vi "monitor INTAKE power curve.vi"() -> ()   [LabVIEW 2023]
uses:
  <vilib>/Rock Robotics/WPI/ThirdParty/REV Robotics/REVLib/Typedef/Spark MAX Parameter ID.ctl
  <vilib>/Rock Robotics/WPI/ThirdParty/REV Robotics/REVLib/Typedef/Spark MAX Parameter Type.ctl
  Global INIT.vi
  Global stack names.vi
panel:
  out "motor rpm":dbl
  out "kVelocity\nConversion":dbl
  out "kPosition\nConversion":dbl
  in  "reset maxes":bool
  out "Power (W)\nMAX":dbl format="%#_13g"
  out "current (A)\nMAX":dbl format="%#_13g"
  out "Temp (F)\nMAX":i8
  out "Monitoring INTAKE motor":T1(graph)
  in  "error in (no error)":errorcluster
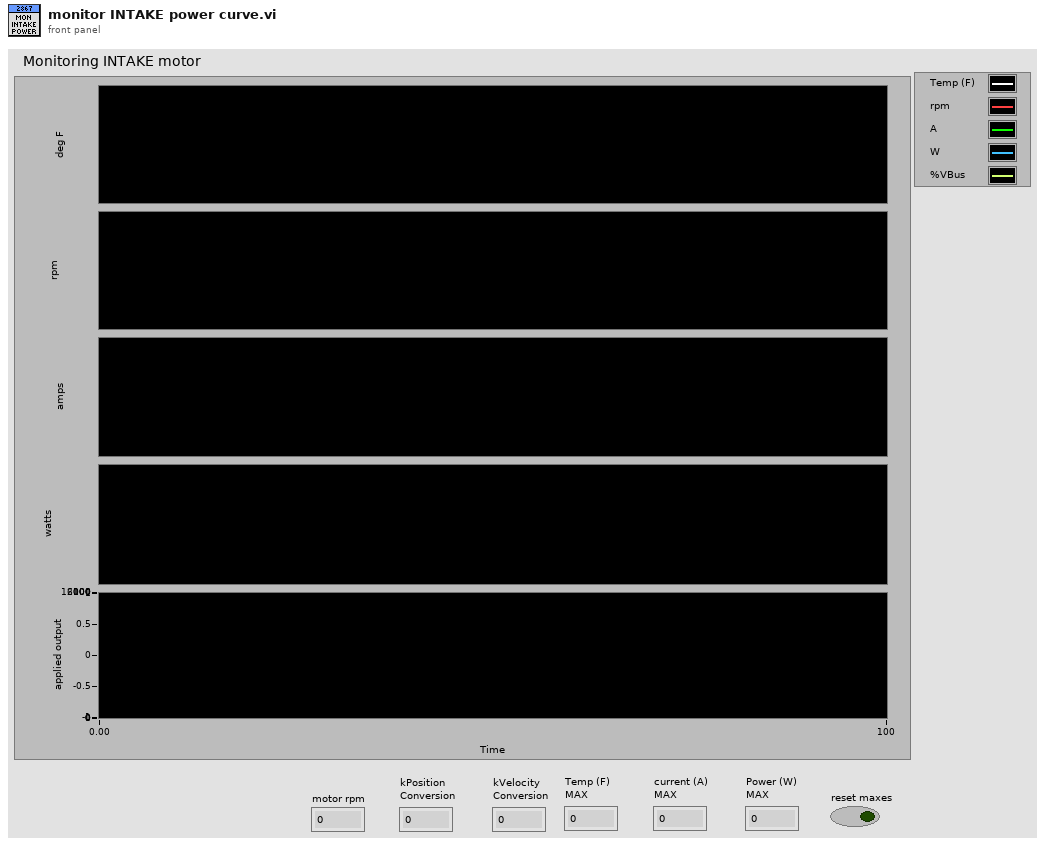
[diagram p1: front panel]
types:
  T1 = cluster{"Motor Temperature":u8, "Sensor Velocity":dbl, "Motor Current":dbl, dbl, "Applied Output":dbl}
  T2 = typedef "Spark MAX Parameter Type.ctl" = enum16{"Signed Int", "Unsigned Int", "Float", "Bool"}
  T3 = typedef "Spark MAX Parameter ID.ctl" = enum16{"kCanID", "kInputMode", "kMotorType", "kCommAdvance", "kSensorType", "kCtrlType", "kIdleMode", "kInputDeadband", "kFeedbackSensorPID0", "kFeedbackSensorPID1", "kPolePairs", "kCurrentChop", "kCurrentChopCycles", "kP_0", "kI_0", "kD_0", "kF_0", "kIZone_0", "kDFilter_0", "kOutputMin_0", "kOutputMax_0", "kP_1", "kI_1", "kD_1", "kF_1", "kIZone_1", "kDFilter_1", "kOutputMin_1", "kOutputMax_1", "kP_2", "kI_2", "kD_2", "kF_2", "kIZone_2", "kDFilter_2", "kOutputMin_2", "kOutputMax_2", "kP_3", "kI_3", "kD_3", "kF_3", "kIZone_3", "kDFilter_3", "kOutputMin_3", "kOutputMax_3", "kInverted", "kOutputRatio", "kSerialNumberLow", "kSerialNumberMid", "kSerialNumberHigh", "kLimitSwitchFwdPolarity", "kLimitSwitchRevPolarity", "kHardLimitFwdEn", "kHardLimitRevEn", "kSoftLimitFwdEn", "kSoftLimitRevEn", "kRampRate", "kFollowerID", "kFollowerConfig", "kSmartCurrentStallLimit", "kSmartCurrentFreeLimit", "kSmartCurrentConfig", "kSmartCurrentReserved", "kMotorKv", "kMotorR", "kMotorL", "kMotorRsvd1", "kMotorRsvd2", "kMotorRsvd3", "kEncoderCountsPerRev", "kEncoderAverageDepth", "kEncoderSampleDelta", "kEncoderInverted", "kEncoderRsvd1", "kClosedLoopVoltageMode", "kCompensatedNominalVoltage", "kSmartMotionMaxVelocity_0", "kSmartMotionMaxAccel_0", "kSmartMotionMinVelOutput_0", "kSmartMotionAllowedClosedLoopError_0", "kSmartMotionAccelStrategy_0", "kSmartMotionMaxVelocity_1", "kSmartMotionMaxAccel_1", "kSmartMotionMinVelOutput_1", "kSmartMotionAllowedClosedLoopError_1", "kSmartMotionAccelStrategy_1", "kSmartMotionMaxVelocity_2", "kSmartMotionMaxAccel_2", "kSmartMotionMinVelOutput_2", "kSmartMotionAllowedClosedLoopError_2", "kSmartMotionAccelStrategy_2", "kSmartMotionMaxVelocity_3", "kSmartMotionMaxAccel_3", "kSmartMotionMinVelOutput_3", "kSmartMotionAllowedClosedLoopError_3", "kSmartMotionAccelStrategy_3", "kIMaxAccum_0", "kSlot3Placeholder1_0", "kSlot3Placeholder2_0", "kSlot3Placeholder3_0", "kIMaxAccum_1", "kSlot3Placeholder1_1", "kSlot3Placeholder2_1", "kSlot3Placeholder3_1", "kIMaxAccum_2", "kSlot3Placeholder1_2", "kSlot3Placeholder2_2", "kSlot3Placeholder3_2", "kIMaxAccum_3", "kSlot3Placeholder1_3", "kSlot3Placeholder2_3", "kSlot3Placeholder3_3", "kPositionConversionFactor", "kVelocityConversionFactor", "kClosedLoopRampRate", "kSoftLimitFwd", "kSoftLimitRev", "kSoftLimitRsvd0", "kSoftLimitRsvd1", "kAnalogPositionConversion", "kAnalogVelocityConversion", "kAnalogAverageDepth", "kAnalogSensorMode", "kAnalogInverted", "kAnalogSampleDelta", "kAnalogRsvd0", "kAnalogRsvd1", "kDataPortConfig", "kAltEncoderCountsPerRev", "kAltEncoderAverageDepth", "kAltEncoderSampleDelta", "kAltEncoderInverted", "kAltEncoderPositionConversion", "kAltEncoderVelocityConversion", "kAltEncoderRsvd0", "kAltEncoderRsvd1", "kHallSensorSampleRate", "kHallSensorAverageDepth", "kNumParameters", "kDutyCyclePositionFactor", "kDutyCycleVelocityFactor", "kDutyCycleInverted", "kDutyCycleSensorMode", "kDutyCycleAverageDepth", "kDutyCycleSampleDelta", "kDutyCycleOffsetv1p6p2", "kDutyCycleRsvd0", "kDutyCycleRsvd1", "kDutyCycleRsvd2", "kPositionPIDWrapEnable", "kPositionPIDMinInput", "kPositionPIDMaxInput", "kDutyCycleZeroCentered", "kDutyCyclePrescalar", "kDutyCycleOffset", "kProductId", "kDeviceMajorVersion", "kDeviceMinorVersion"}
  T4 = typedef "ctrl swerve motor.ctl" = cluster{"description":string, "MOTOR SELECT":T5, "Installed?":bool, "CAN ID":u8, "refnum name":string, "Invert":bool, "Idle Mode":T6, "Current limiting":T7, "MOTOR PIDF coefficients":T8, "gear ratio":dbl}
  T5 = typedef "ctrl MOTOR SELECT.ctl" = i16
  T6 = typedef "Spark MAX Idle Mode.ctl" = enum16{"Coast", "Brake"}
  T7 = typedef "ctrl Spark MAX current limiting.ctl" = cluster{"Linearized":bool, "Free Speed (A)":dbl, "Primay (A)":dbl, "Limit RPM (0)":u32}
  T8 = typedef "ctrl motor PIDF coefficients.ctl" = cluster{"PIDF":cluster{"P Gain":dbl, "I Gain":dbl, "D Gain":dbl, "F Gain":dbl, "I Zone":dbl, "Min Output":dbl, "Max Output":dbl}, "Smart Motion":T9}
  T9 = typedef "Spark MAX Smart Motion Parameters.ctl" = cluster{"Max Velocity":dbl, "Max Acceleration":dbl, "Minimum Velocity Output":dbl, "Allowed Closed Loop Error":dbl}
  T10 = typedef "WPI_MotorControlDeviceRef.ctl" = cluster{"DeviceStatus":errorcluster, "Type":T11, "PWM":cluster{"PWM Channel":T12, "DeadBand":T13}, "CAN":cluster{"Device Number":u8, "SetOutput VI Ref":variant, "GetOutput VI Ref":variant, "Enable VI Ref":variant, "Disable VI Ref":variant, "Data":variant}, "Invert":bool, "DIO PWM":cluster{"PWM \"Enable\" Channel":T12, "DIOChannel":T14, "PWM Rate":dbl}}
  T11 = typedef "WPI_MotorControlType.ctl" = enum16{"PWM", "CAN", "DIO PWM"}
  T12 = typedef "FPGA_DIOPWMChannel.ctl" = enum8{"PWM 0", "PWM 1", "PWM 2", "PWM 3", "PWM 4", "PWM 5", "PWM 6", "PWM 7", "PWM 8", "PWM 9", "PWM MXP 0", "PWM MXP 1", "PWM MXP 2", "PWM MXP 3", "PWM MXP 4", "PWM MXP 5", "PWM MXP 6", "PWM MXP 7", "PWM MXP 8", "PWM MXP 9", "Invalid"}
  T13 = typedef "WPI_PWMDeadband.ctl" = cluster{"Name":string, "maxPositivePwm":i32, "minPositivePwm":i32, "centerPwm":i32, "maxNegativePwm":i32, "minNegativePwm":i32, "angularRange":u16}
  T14 = typedef "FPGA_DIOChannel.ctl" = enum8{"DIO 0", "DIO 1", "DIO 2", "DIO 3", "DIO 4", "DIO 5", "DIO 6", "DIO 7", "DIO 8", "DIO 9", "DIO MXP 0", "DIO MXP 1", "DIO MXP 2", "DIO MXP 3", "DIO MXP 4", "DIO MXP 5", "DIO MXP 6", "DIO MXP 7", "DIO MXP 8", "DIO MXP 9", "DIO MXP 10", "DIO MXP 11", "DIO MXP 12", "DIO MXP 13", "DIO MXP 14", "DIO MXP 15", "SPI Port CS1", "SPI Port CS2", "SPI Port CS3", "SPI Port MISO", "SPI Port MOSI", "Invalid"}
  T15 = typedef "Spark MAX Status 1 Frame.ctl" = cluster{"Sensor Velocity":dbl, "Motor Temperature":u8, "Motor Voltage":dbl, "Motor Current":dbl, "Timestamp":u32}
  T16 = cluster{"Motor Temperature":u8, dbl, "Motor Current":dbl, dbl, "Applied Output":dbl}
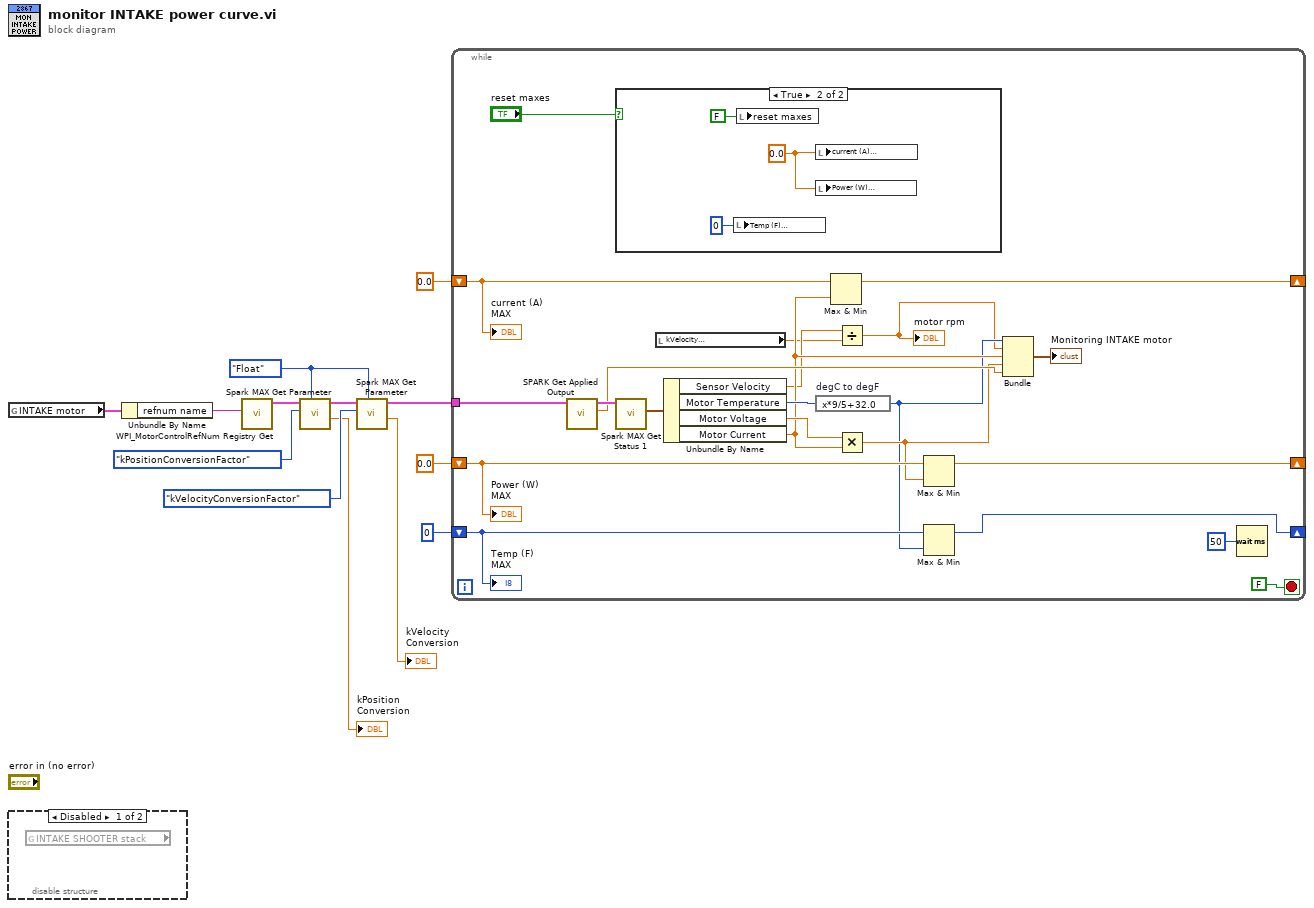
[diagram p0: block diagram]
diagram:
  w1 = Spark_MAX_Parameter_Type."Float" ("Expected Type")
  n1 = global read "Global INIT.vi" "INTAKE motor"() -> (w13:T4)
  n2 = disable-structure shown="Disabled" {
    frame Disabled {
      n3 = global read "Global stack names.vi" "INTAKE SHOOTER stack"() -> ()  [unwired: 1 out]
    }
    frame Enabled {
    }
  }
  n4 = Unbundle By Name(w13) -> ("refnum name"=w12:string)
  n5 = call <vilib>:"WPI_MotorControlRefNum Registry Get.vi"("refnum name"=w12) -> ("MotorControlDevRef"=w8:T10)  [unwired: 9 in, 1 out]
  n6 = call <vilib>:"Spark MAX Get Parameter.vi"("Expected Type"=w1, "Parameter ID in"=Spark_MAX_Parameter_ID."kPositionConversionFactor" ("Parameter ID"), "MotorControlDeviceRef in"=w8) -> ("float"=→"kPosition\nConversion":dbl, "MotorControlDeviceRef"=w7:T10)  [unwired: 3 in, 4 out]
  n7 = call <vilib>:"Spark MAX Get Parameter.vi"("Expected Type"=w1, "Parameter ID in"=Spark_MAX_Parameter_ID."kVelocityConversionFactor" ("Parameter ID"), "MotorControlDeviceRef in"=w7) -> ("float"=→"kVelocity\nConversion":dbl, "MotorControlDeviceRef"=w6:T10)  [unwired: 3 in, 4 out]
  n8 = while {
    tunnel: w6 -> [w32]
    shift-right: [w24] -> _
    shift-left: 0.0 ("Power (W)\nMAX 2") -> [w23]
    shift-right: [w21] -> _
    shift-left: 0.0 ("current (A)\nMAX 2") -> [w25]
    shift-right: [w19] -> _
    shift-left: i8 0 ("Temp (F)\nMAX 2") -> [w26]
    stop <- FALSE stop-if-true
    n9 = call <vilib>:"SPARK Get Applied Output.vi"("MotorControlDevRef in"=w32) -> ("Applied Output"=w27:dbl, "MotorControlDevRef out"=w34:T10)  [unwired: 7 in, 2 out]
    n10 = case shown="True" "reset maxes" {
      frame False {
      }
      frame True {
        w37 = 0.0 ("Power (W)\nMAX")
        n11 = local write "Temp (F)\nMAX"(i8 0 ("Temp (F)\nMAX")) -> ()
        n12 = local write "reset maxes"(FALSE ("reset maxes")) -> ()
        n13 = local write "current (A)\nMAX"(w37) -> ()
        n14 = local write "Power (W)\nMAX"(w37) -> ()
      }
    }
    n15 = call <vilib>:"Spark MAX Get Status 1.vi"("MotorControlDevRef"=w34) -> ("Status 1"=w35:T15)  [unwired: 7 in, 3 out]
    n16 = local read "kVelocity\nConversion"() -> (w15:dbl)
    n17 = Unbundle By Name(w35) -> ("Sensor Velocity"=w16:dbl, "Motor Temperature"=w28:u8, "Motor Voltage"=w33:dbl, "Motor Current"=w20:dbl)
    n18 = expression code="x*9/5+32.0" "degC to degF"(w28) -> (w18:u8)
    n19 = Max & Min(x=w25, y=w20) -> (max(x,y)=w21:dbl)  [unwired: 1 out]
    n20 = Divide(x=w16, y=w15) -> (x/y=w14:dbl)
    "motor rpm" <- w14
    n21 = Multiply(x=w33, y=w20) -> (x*y=w22:dbl)
    n22 = Max & Min(x=w23, y=w22) -> (max(x,y)=w24:dbl)  [unwired: 1 out]
    n23 = Max & Min(x=w26, y=w18) -> (max(x,y)=w19:u8)  [unwired: 1 out]
    n24 = Bundle("Motor Temperature"=w18, w14, "Motor Current"=w20, w22, "Applied Output"=w27) -> (→"Monitoring INTAKE motor":T16)  [unwired: 1 in]
    n25 = Wait (ms)(milliseconds to wait=u32 50) -> ()  [unwired: 1 out]
    "Temp (F)\nMAX" <- w26
    "current (A)\nMAX" <- w25
    "Power (W)\nMAX" <- w23
  }
